vi "CAN Loop.vi"() -> ()   [LabVIEW 2018]
uses:
  Type Defs/Controller Names.ctl
  Type Defs/CAN Mode.ctl
panel:
  out "CAN CMD":dbl
  in  "Controller Type:":T1
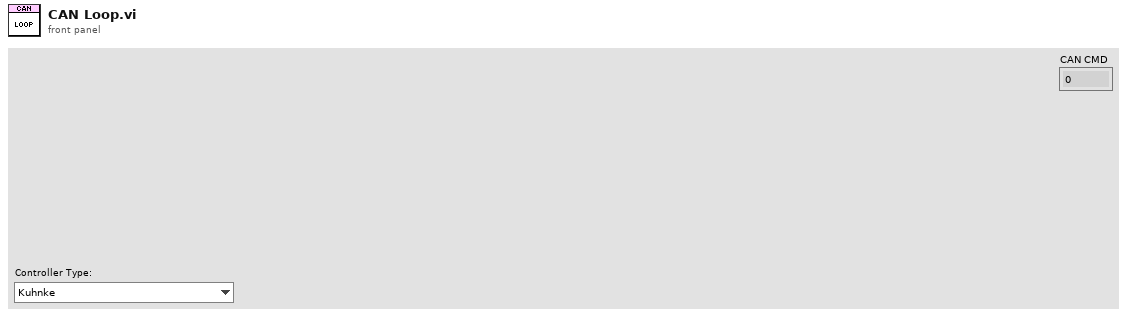
[diagram p1: front panel]
types:
  T1 = typedef "Controller Names.ctl" = enum16{"Kuhnke", "Helbako BLDC", "Conti", "Hella BLDC OL PWM", "Hella BLDC Turbine OL PWM", "Hella BLDC Pressure", "Helbako (old)", "TI PWM", "PSA", "Hella Gas", "Hella Diesel", "8 Comm", "10 Comm", "8 Comm Hella", "10 Comm Hella", "8 Comm Omron", "10 Comm Omron", "8 Comm Nissan", "10 Comm Nissan"}
  T2 = typedef "CAN Mode.ctl" = enum16{"Init", "Read", "Write", "Close"}
  T3 = cluster{"Pump 1":bool, "Pump 2":bool, "Pump 3":bool, "Pump 4":bool, "Pump 5":bool, "Pump 6":bool}
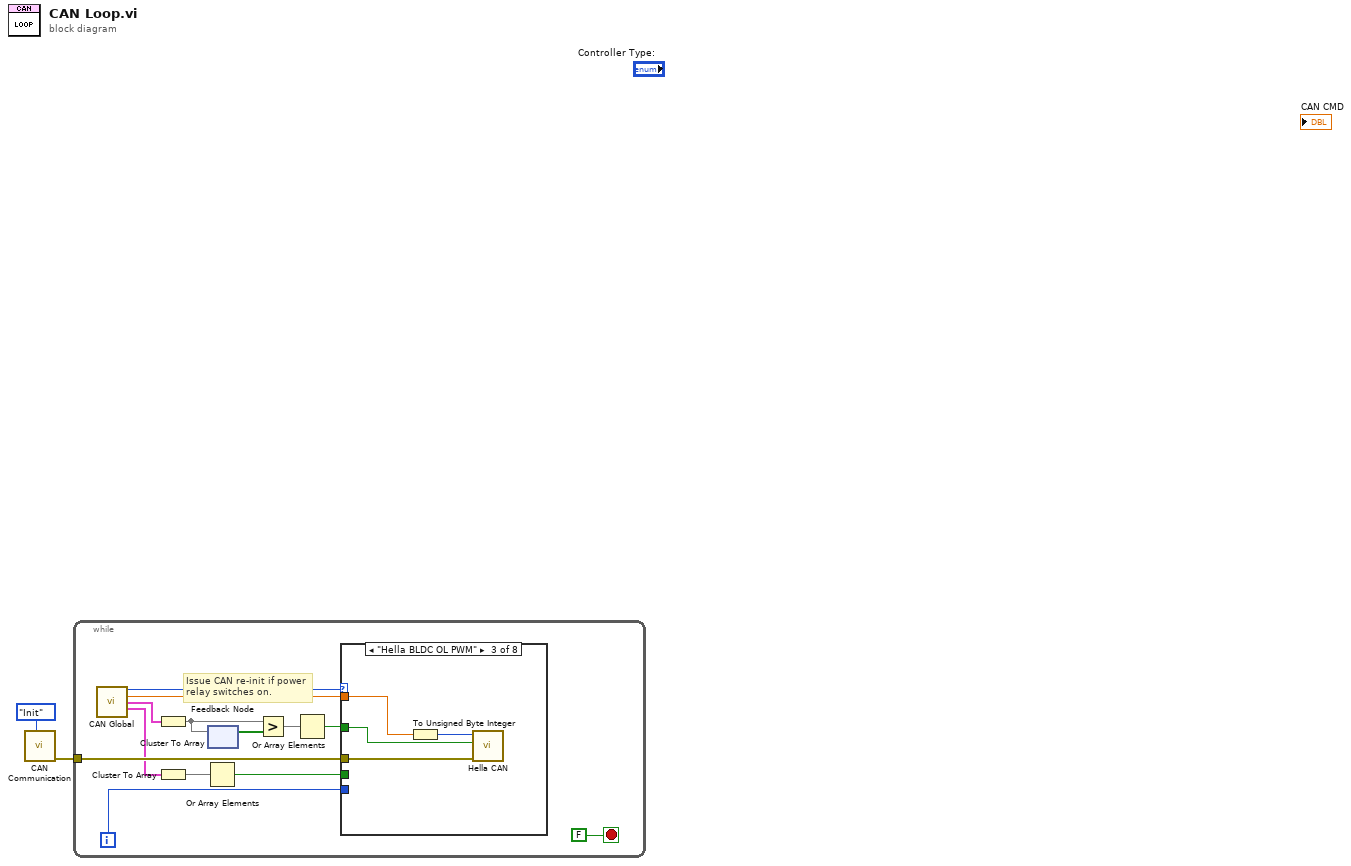
[diagram p0: block diagram]
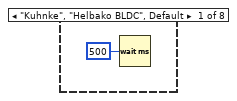
[diagram p2: hidden frame]
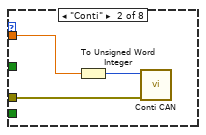
[diagram p3: hidden frame]
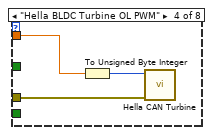
[diagram p4: hidden frame]
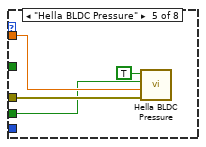
[diagram p5: hidden frame]
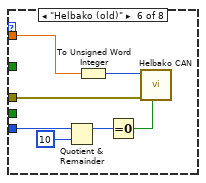
[diagram p6: hidden frame]
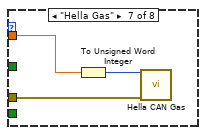
[diagram p7: hidden frame]
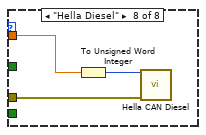
[diagram p8: hidden frame]
diagram:
  n1 = call "CAN Communication.vi"("CAN Mode"=CAN_Mode."Init") -> ("Error OUT"=w1:errorcluster)  [unwired: 9 in, 1 out]
  n2 = while {
    tunnel: w1 -> [w14]
    i -> [w13]
    stop <- FALSE stop-if-true
    # "Issue CAN re-init if power\nrelay switches on."
    n3 = call "CAN Global.vi"() -> ("Controller Type OUT"=w12:T1, "CAN Cmd OUT"=w6:dbl, "Power Relay OUT"=w8:T3, "Ignition Relay OUT"=w4:T3)  [unwired: 12 in]
    n4 = Cluster To Array(cluster=w8) -> (array=w11:bool[])
    n5 = Cluster To Array(cluster=w4) -> (array=w5:bool[])
    n6 = Or Array Elements(Boolean array=w5) -> (logical OR=w3:bool)
    n7 = feedback #1() -> (w10:bool[])  [unwired: 1 in]
    n8 = feedback-in #1(w11) -> ()
    n9 = Greater?(x=w11, y=w10) -> (0:w9:bool[])
    n10 = Or Array Elements(Boolean array=w9) -> (logical OR=w7:bool)
    n11 = case shown="\"Hella BLDC OL PWM\"" w12 {
      tunnel: w14 -> [_ w19 w23 w24 w30 w35 w39 w43]
      tunnel: w6 -> [_ w18 w22 w26 w29 w37 w40 w41]
      tunnel: w13 -> [_ _ _ _ _ w34 _ _]
      tunnel: w7 -> [_ _ w20 _ _ _ _ _]
      tunnel: w3 -> [_ _ _ _ w27 _ _ _]
      frame "Kuhnke", "Helbako BLDC", Default {
        n12 = Wait (ms)(milliseconds to wait=u32 500) -> ()  [unwired: 1 out]
      }
      frame "Conti" {
        n13 = To Unsigned Word Integer(number=w18) -> (unsigned 16bit integer=w17:u16)
        n14 = call "Conti CAN.vi"("Error IN"=w19, "CMD"=w17) -> ()  [unwired: 9 in, 1 out]
      }
      frame "Hella BLDC OL PWM" {
        n15 = To Unsigned Byte Integer(number=w22) -> (unsigned 8bit integer=w21:u8)
        n16 = call "Hella CAN.vi"("Error IN"=w23, "Re-Init CAN"=w20, "CMD"=w21) -> ()  [unwired: 8 in, 1 out]
      }
      frame "Hella BLDC Turbine OL PWM" {
        n17 = To Unsigned Byte Integer(number=w26) -> (unsigned 8bit integer=w25:u8)
        n18 = call "Hella CAN Turbine.vi"("Error IN"=w24, "CMD"=w25) -> ()  [unwired: 9 in, 1 out]
      }
      frame "Hella BLDC Pressure" {
        n19 = call "Hella BLDC Pressure.vi"("Error IN"=w30, "Pressure"=w29, "IGN"=w27, "Run?"=TRUE) -> ()  [unwired: 7 in, 1 out]
      }
      frame "Helbako (old)" {
        n20 = Quotient & Remainder(x=w34, y=10) -> (x-y*floor(x/y)=w32:i32)  [unwired: 1 out]
        n21 = To Unsigned Word Integer(number=w37) -> (unsigned 16bit integer=w36:u16)
        n22 = Equal To 0?(x=w32) -> (x = 0?=w31:bool)
        n23 = call "Helbako CAN.vi"("Split-timer"=w31, "Error IN"=w35, "CMD"=w36) -> ()  [unwired: 8 in, 1 out]
      }
      frame "Hella Gas" {
        n24 = To Unsigned Word Integer(number=w40) -> (unsigned 16bit integer=w38:u16)
        n25 = call "Hella CAN Gas.vi"("Pressure Command (kPa)"=w38, "Error In"=w39) -> ()  [unwired: 12 in, 2 out]
      }
      frame "Hella Diesel" {
        n26 = To Unsigned Word Integer(number=w41) -> (unsigned 16bit integer=w42:u16)
        n27 = call "Hella CAN Diesel.vi"("Command (kPa)"=w42, "Error In"=w43) -> ()  [unwired: 13 in, 1 out]
      }
    }
  }
